vi "Match Substring Unicode.vi"(6 "Offset (0)":i32, 7 "Substring (U16) [ ]":u16[](array[numeric]), 9 "String (U16) [ ]":u16[](array[numeric])) -> (0 "offset past match":i32=-1, 1 "after substring":u16[](array[numeric]), 2 "match substring":u16[](array[numeric]), 3 "before substring":u16[](array[numeric]))   [LabVIEW 2019, in "Exaprom PDF.lvlib"]
doc: "Version 1.1\nDeveloped by Jean-Marc Simard\nCopyright © 2012, Exaprom Inc.\nAll rights reserved.\nLicense: BSD\n\nWith iTextSharp 4.1.6 (http://itextsharp.sourceforge.net)\nunder Mozilla Public License Version 1.1\n(http://www.mozilla.org/MPL/MPL-1.1.html)"
uses:
  Exaprom PDF.lvlib
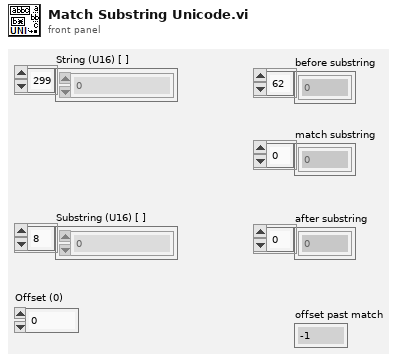
[diagram p1: front panel]
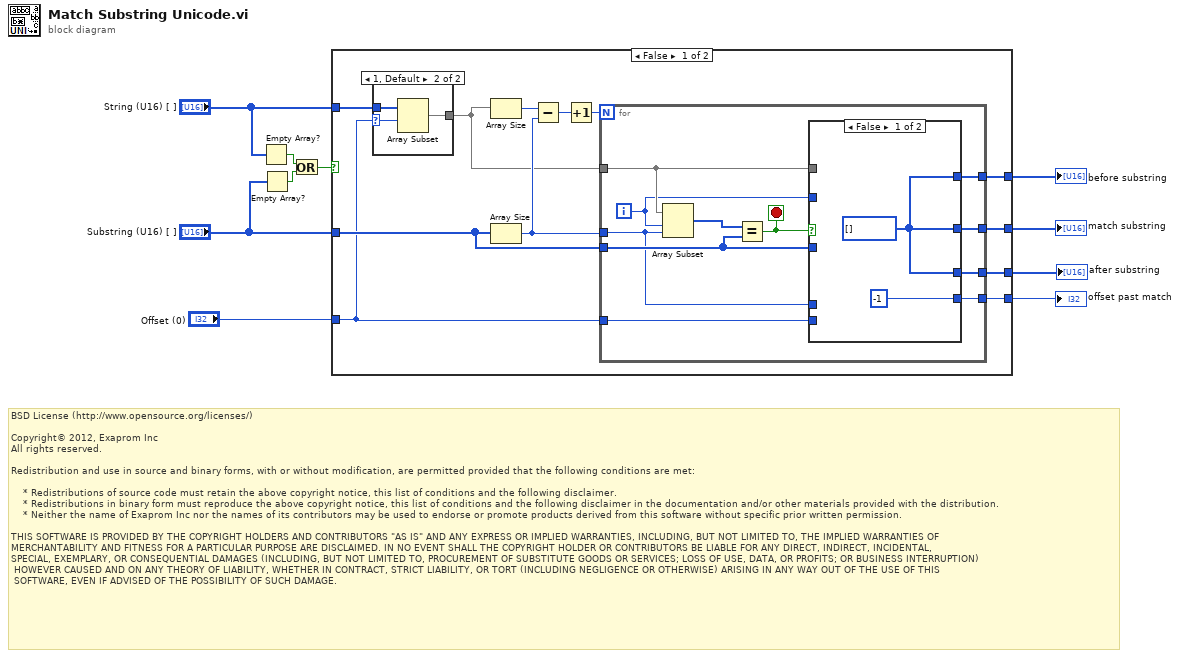
[diagram p0: block diagram]
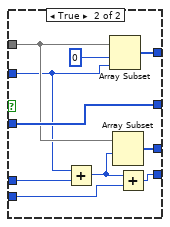
[diagram p3: hidden frame]
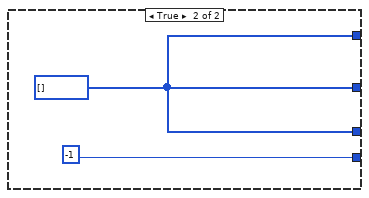
[diagram p4: hidden frame]
diagram:
  # "BSD License (http://www.opensource.org/licenses/)\n\nCopyright© 2012, Exaprom Inc\nAll rights reserved.\n\nRedistribution and use in source and binary forms, with or without modification, are permitted provided that the following conditions are met:\n\n    * Redistributions of source code must retain the above copyright notice, this list of conditions and the following disclaimer.\n    * Redistributions in binary form must reproduce the above copyright notice, this list of conditions and the following disclaimer in the documentation and/or other materials provided with the distribution.\n    * Neither the name of Exaprom Inc nor the names of its contributors may be used to endorse or promote products derived from this software without specific prior written permission.\n\nTHIS SOFTWARE IS PROVIDED BY THE COPYRIGHT HOLDERS AND CONTRIBUTORS \"AS IS\" AND ANY EXPRESS OR IMPLIED WARRANTIES, INCLUDING, BUT NOT LIMITED TO, THE IMPLIED WARRANTIES OF \nMERCHANTABILITY AND FITNESS FOR A PARTICULAR PURPOSE ARE DISCLAIMED. IN NO EVENT SHALL THE COPYRIGHT HOLDER OR CONTRIBUTORS BE LIABLE FOR ANY DIRECT, INDIRECT, INCIDENTAL,\nSPECIAL, EXEMPLARY, OR CONSEQUENTIAL DAMAGES (INCLUDING, BUT NOT LIMITED TO, PROCUREMENT OF SUBSTITUTE GOODS OR SERVICES; LOSS OF USE, DATA, OR PROFITS; OR BUSINESS INTERRUPTION)\n HOWEVER CAUSED AND ON ANY THEORY OF LIABILITY, WHETHER IN CONTRACT, STRICT LIABILITY, OR TORT (INCLUDING NEGLIGENCE OR OTHERWISE) ARISING IN ANY WAY OUT OF THE USE OF THIS\n SOFTWARE, EVEN IF ADVISED OF THE POSSIBILITY OF SUCH DAMAGE."
  n1 = Empty Array?(array="String (U16) [ ]") -> (empty?=w5:bool)
  n2 = Empty Array?(array="Substring (U16) [ ]") -> (empty?=w4:bool)
  n3 = Or(x=w5, y=w4) -> (x .or. y?=w6:bool)
  n4 = case shown="False" w6 {
    tunnel: [w18 w50] -> w10
    tunnel: [w17 w50] -> w9
    tunnel: [w16 w50] -> w8
    tunnel: [w15 -1 ("index")] -> w7
    tunnel: "String (U16) [ ]" -> [w13 _]
    tunnel: "Substring (U16) [ ]" -> [w14 _]
    tunnel: "Offset (0)" -> [w11 _]
    frame False {
      n5 = case shown="1, Default" w11 {
        selector: w11 -> [_ w24]
        tunnel: w13 -> [w23 w26]
        tunnel: [w23 w25] -> w12
        frame 0 {
        }
        frame 1, Default {
          n6 = Array Subset(array=w26, index=w24) -> (w25:u16[])  [unwired: 1 in]
        }
      }
      n7 = Array Size(array=w12) -> (size(s)=w22:i32)
      n8 = Array Size(array=w14) -> (size(s)=w20:i32)
      n9 = Subtract(x=w22, y=w20) -> (x-y=w21:i32)
      n10 = Increment(x=w21) -> (x+1=w19:i32)
      n11 = for {
        N: w19 -> [_]
        tunnel: w12 -> [w35]
        tunnel: w14 -> [w32]
        tunnel: w20 -> [w28]
        tunnel: [w33] -> w18
        tunnel: [w31] -> w17
        tunnel: [w30] -> w16
        tunnel: [w29] -> w15
        tunnel: w11 -> [w27]
        i -> [w34]
        stop <- w36 stop-if-true
        n12 = Array Subset(array=w35, index=w34, length=w28) -> (w37:u16[])
        n13 = Equal?(x=w37, y=w32) -> (x = y?=w36:bool)
        n14 = case shown="False" w36 {
          tunnel: w35 -> [_ w46]
          tunnel: w34 -> [_ w44]
          tunnel: [w39 w48] -> w33
          tunnel: [w39 w47] -> w31
          tunnel: w32 -> [_ w47]
          tunnel: [w39 w45] -> w30
          tunnel: [-1 ("index") w43] -> w29
          tunnel: w28 -> [_ w40]
          tunnel: w27 -> [_ w41]
          frame False {
            w39 = u16[] []
          }
          frame True {
            n15 = Add(x=w44, y=w40) -> (x+y=w42:i32)
            n16 = Array Subset(array=w46, index=0, length=w44) -> (w48:u16[])
            n17 = Array Subset(array=w46, index=w42) -> (w45:u16[])  [unwired: 1 in]
            n18 = Add(x=w42, y=w41) -> (x+y=w43:i32)
          }
        }
      }
    }
    frame True {
      w50 = u16[] []
    }
  }
  "before substring" <- w10
  "match substring" <- w9
  "after substring" <- w8
  "offset past match" <- w7
